vi "Fill FN - Post-Fill Wait (SubVI).vi"(0 "Signals IN":T1={"Dispense"=FALSE, "Fill"=FALSE, "Spray"=FALSE, "Drain"=TRUE, "Complete"=FALSE, "Fill Error"=FALSE, "Disp. Error"=FALSE, "Fill Timeout"=FALSE, "Disp. Timeout"=FALSE, "Purge"=TRUE}, 1 "Values IN":T2 {"Drain Time (s)" format="%.2f"; "Drain Rate (g/sec)" format="%.2f"}, 2 "Measured Mass (g)":dbl(knob) scale=0.0..1000.0, 5 "Fill Case Change?":bool, 9 "Full \nSettle Time (s)":dbl) -> (14 "Signals OUT":T1={"Dispense"=FALSE, "Fill"=FALSE, "Spray"=FALSE, "Drain"=TRUE, "Complete"=FALSE, "Fill Error"=FALSE, "Disp. Error"=FALSE, "Fill Timeout"=FALSE, "Disp. Timeout"=FALSE, "Purge"=TRUE}, 15 "Values OUT":T2, 19 "Case Complete":bool)   [LabVIEW 2011]
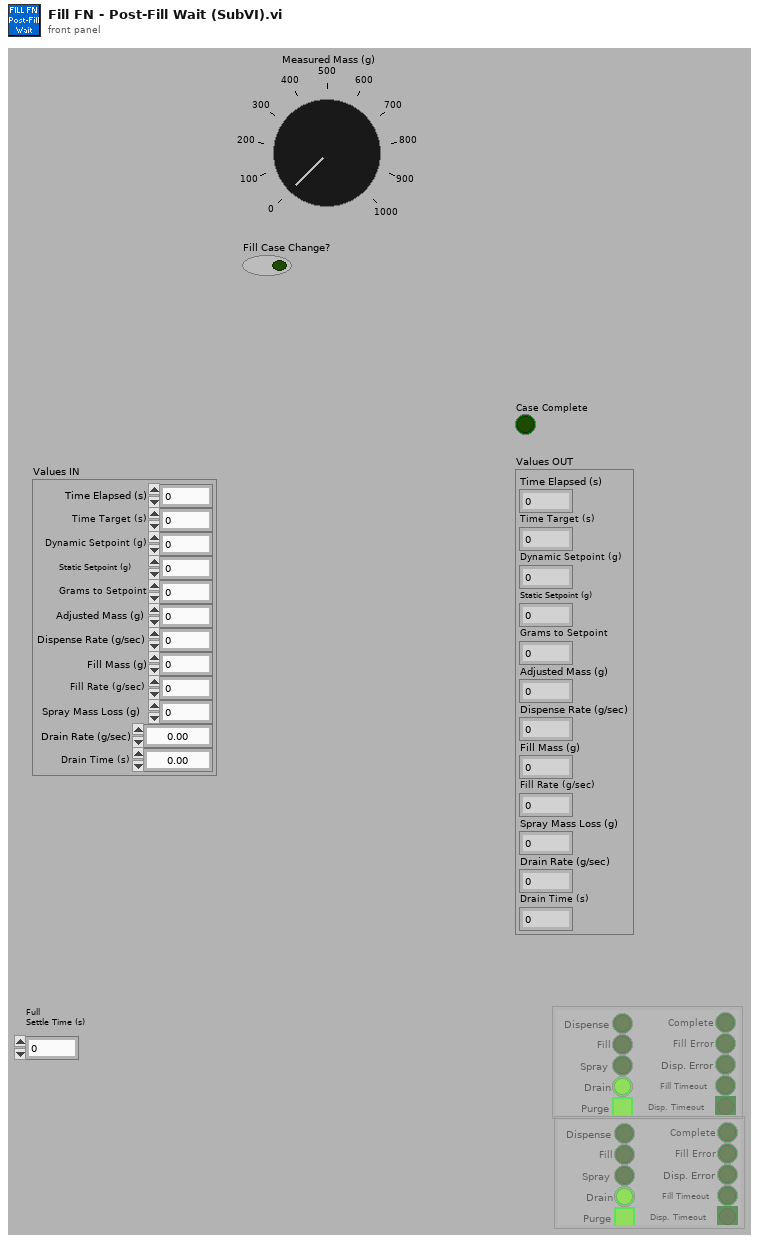
[diagram p1: front panel]
types:
  T1 = cluster{"Dispense":bool, "Fill":bool, "Spray":bool, "Drain":bool, "Complete":bool, "Fill Error":bool, "Disp. Error":bool, "Fill Timeout":bool, "Disp. Timeout":bool, "Purge":bool}
  T2 = cluster{"Time Elapsed (s)":dbl, "Time Target (s)":dbl, "Dynamic Setpoint (g)":dbl, "Static Setpoint (g)":dbl, "Grams to Setpoint":dbl, "Adjusted Mass (g)":dbl, "Dispense Rate (g/sec)":dbl, "Fill Mass (g)":dbl, "Fill Rate (g/sec)":dbl, "Spray Mass Loss (g)":dbl, "Drain Rate (g/sec)":dbl, "Drain Time (s)":dbl}
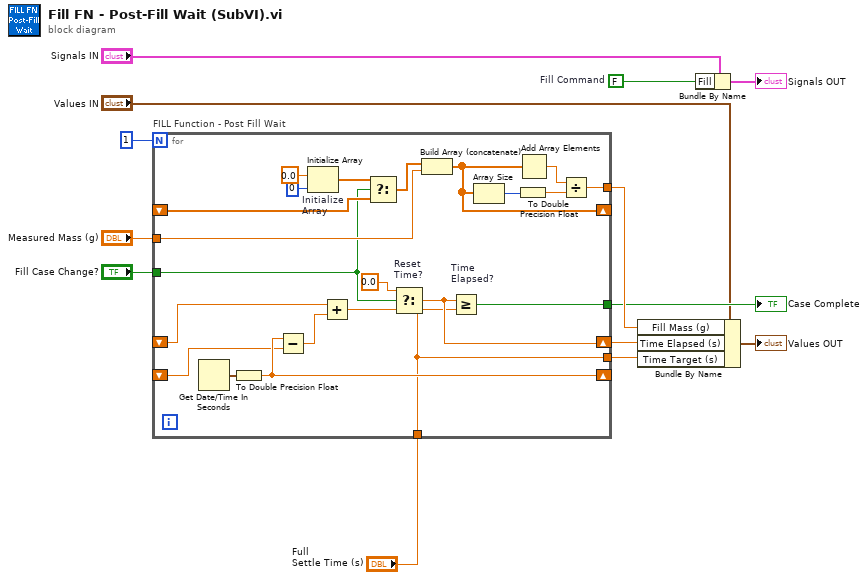
[diagram p0: block diagram]
diagram:
  w8 = FALSE  # Fill Command
  n1 = for "FILL Function - Post Fill Wait" {
    N: 1 -> [_]
    shift-right: [w34] -> _
    shift-left: _ -> [w33]
    shift-right: [w28] -> w10
    shift-left: _ -> [w31]
    tunnel: "Measured Mass (g)" -> [w18]
    tunnel: "Fill Case Change?" -> [w17]
    tunnel: [w16] -> w13
    shift-right: [w25] -> _
    shift-left: _ -> [w19]
    tunnel: [w14] -> w11
    tunnel: [w15] -> w12
    tunnel: "Full \nSettle Time (s)" -> [w14]
    n2 = Get Date/Time In Seconds() -> (seconds since 1Jan1904=w35:timestamp)
    n3 = To Double Precision Float(number=w35) -> (double precision float=w34:dbl)
    n4 = Subtract(x=w34, y=w33) -> (x-y=w30:dbl)
    n5 = Initialize Array "Initialize\nArray"(0.0 ("Measured Mass (g)"), 0 ("dimension size")) -> (w21:dbl[])
    n6 = Add(x=w31, y=w30) -> (x+y=w32:dbl)
    n7 = Select(t=w21, s=w17, f=w19) -> (s? t:f=w20:dbl[])
    n8 = Select "Reset\nTime?"(t=0.0, s=w17, f=w32) -> (s? t:f=w28:dbl)
    n9 = Build Array (concatenate)(w20, w18) -> (w25:dbl[])
    n10 = Greater Or Equal? "Time\nElapsed?"(x=w28, y=w14) -> (x >= y?=w15:bool)
    n11 = Array Size(array=w25) -> (size(s)=w23:i32)
    n12 = To Double Precision Float(number=w23) -> (double precision float=w22:dbl)
    n13 = Add Array Elements(numeric array=w25) -> (sum=w24:dbl)
    n14 = Divide(x=w24, y=w22) -> (x/y=w16:dbl)
  }
  "Case Complete" <- w12
  n15 = Bundle By Name(cluster="Values IN", "Fill Mass (g)"=w13, "Time Elapsed (s)"=w10, "Time Target (s)"=w11) -> (→"Values OUT":T2)
  n16 = Bundle By Name(cluster="Signals IN", "Fill"=w8) -> (→"Signals OUT":T1)
